vi "MENU_Alarms.vi"(4 "Seconds Very High field alarm":sgl=1.0 caption="Duration sec." min=0 max=1800 format="%#_2f", 5 "Very High field alarm":sgl=5.0 caption="Setpoint" min=1 max=20 format="%_2f", 6 "Seconds High field alarm":sgl=1.0 caption="Duration sec." min=0 max=1800 format="%#_2f", 7 "High field alarm":sgl=0.5 caption="Setpoint" min=0.5 max=20 format="%_2f") -> (0 "Seconds Very High field alarm 2":sgl=1.0 caption="Duration sec." format="%#_1f", 1 "Very High field alarm 2":sgl=5.0 caption="Setpoint" format="%#_1f", 2 "Seconds High field alarm 2":sgl=1.0 caption="Duration sec." format="%#_1f", 3 "High field alarm 2":sgl=1.0 caption="Setpoint" format="%#_1f")   [LabVIEW 2010]
panel:
  in  "Close":bool
  # "ALARMS"
  # "High Field"
  # "Very High Field"
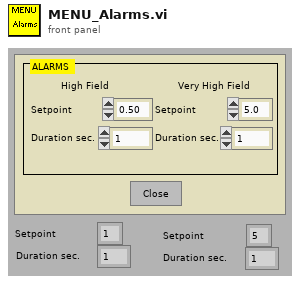
[diagram p1: front panel]
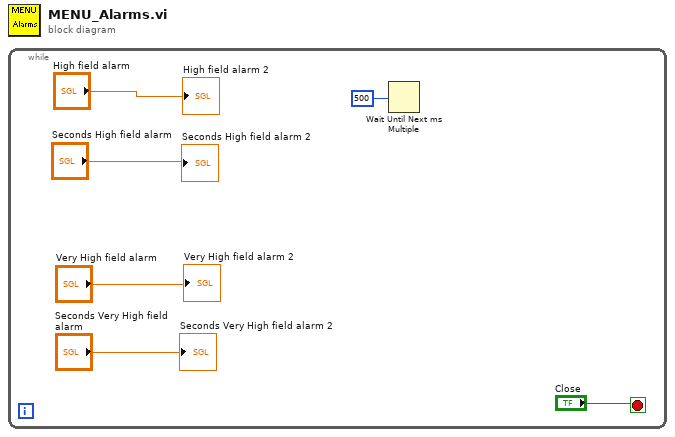
[diagram p0: block diagram]
diagram:
  n1 = while {
    stop <- "Close" stop-if-true
    n2 = Wait Until Next ms Multiple(millisecond multiple=500) -> ()  [unwired: 1 out]
    "High field alarm 2" <- "High field alarm"
    "Seconds High field alarm 2" <- "Seconds High field alarm"
    "Very High field alarm 2" <- "Very High field alarm"
    "Seconds Very High field alarm 2" <- "Seconds Very High field alarm"
  }
